vi "respond to response.vi"(8 "error in (no error)":errorcluster caption="Fehler (Eingang, kein Fehler)", 10 "?":T1={"commandlist"="", "line"=0, "last response"="", "timeout"=0, "wait"=0, "erfolgreich"=FALSE, "next state"=enum."Start", "Zustand"=enum."starting"}, 11 "HF-Felder Eingang":refnum<class "HF-Felder.lvclass"> caption="DNL_LabVIEW Object in") -> (0 "error out":errorcluster caption="Fehler (Ausgang)", 1 "read again?":bool, 2 "?":T1={"commandlist"="", "line"=0, "last response"="", "timeout"=0, "wait"=0, "erfolgreich"=FALSE, "next state"=enum."Start", "Zustand"=enum."starting"}, 3 "HF-Felder Ausgang":refnum<class "HF-Felder.lvclass"> caption="DNL_LabVIEW Object out")   [LabVIEW 2013, in "HF-Felder.lvclass"]
uses:
  HF-Felder.lvclass
  Main/controls/TestData.ctl
  Main/controls/TestStates.ctl
  Main/controls/generalTestStates.ctl
  lib/EMV-Test.lvlib
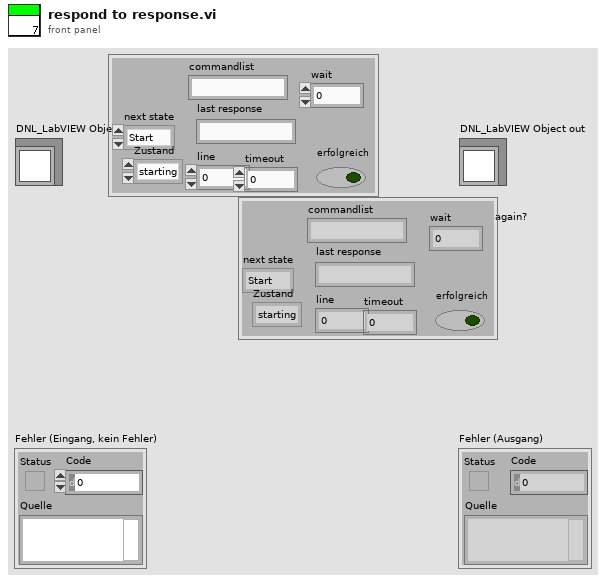
[diagram p1: front panel]
types:
  T1 = typedef "EMV-Test.lvlib/TestData.ctl" = cluster{"commandlist":string, "line":i32, "last response":string, "timeout":i32, "wait":u32, "erfolgreich":bool, "next state":T2, "Zustand":T3}
  T2 = typedef "EMV-Test.lvlib/TestStates.ctl" = enum16{"check for pressed Buttons", "Custom Action 1", "Custom Action 2", "pause", "vorgefertigter Test", "manueller Test", "respond to response", "error", "Start", "Initialise", "evaluate line", "wait for Response", "wait", "catch error", "close Connection", "end"}
  T3 = typedef "generalTestStates.ctl" = enum16{"paused", "starting", "waiting", "running", "finished"}
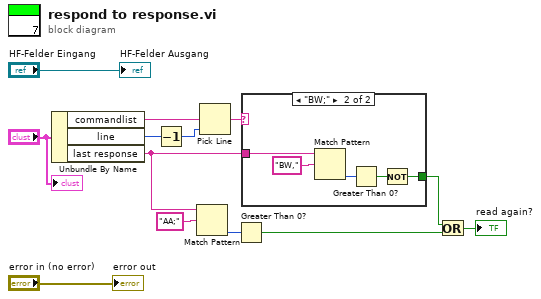
[diagram p0: block diagram]
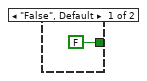
[diagram p2: hidden frame]
diagram:
  n1 = Unbundle By Name("?") -> ("commandlist"=w4:string, "line"=w3:i32, "last response"=w2:string)
  n2 = Decrement(x=w3) -> (x-1=w5:i32)
  n3 = Match Pattern(string=w2, regular expression="AA;") -> (offset past match=w10:i32)  [unwired: 1 in, 3 out]
  n4 = Pick Line(multi-line string=w4, line index=w5) -> (output string=w9:string)  [unwired: 1 in]
  n5 = Greater Than 0?(x=w10) -> (x > 0?=w7:bool)
  n6 = case shown="\"BW;\"" w9 {
    tunnel: w2 -> [_ w17]
    tunnel: [FALSE w15] -> w8
    frame "False", Default {
    }
    frame "BW;" {
      n7 = Match Pattern(string=w17, regular expression="BW,") -> (offset past match=w19:i32)  [unwired: 1 in, 3 out]
      n8 = Greater Than 0?(x=w19) -> (x > 0?=w16:bool)
      n9 = Not(x=w16) -> (.not. x?=w15:bool)
    }
  }
  n10 = Or(x=w8, y=w7) -> (x .or. y?=→"read again?":bool)
  "error out" <- "error in (no error)"
  "HF-Felder Ausgang" <- "HF-Felder Eingang"
  "?" <- "?"
